vi "main_file.vi"() -> ()   [LabVIEW 2015]
uses:
  support VIs/User Event - Stop/User Event - Stop.lvlib
  support VIs/Message Queue/Message Queue.lvlib
  support VIs/Message Queue/Enqueue Message (Single).vi
  Type Definitions/DLTS_user_inputs.ctl
  Type Definitions/Tabs.ctl
  Type Definitions/Technique_selector.ctl
panel:
  out "Tabs 2":T1
  in  "Tabs":T1
  out "Cluster 2":T2
  in  "DLTS user inputs":T3 {"Delay time (ms)" format="%#_4p"; "# Windows" format="%#_4p"; "min window length (ms)" format="%#_4p"; "Pulse width (ms)" format="%#_4p"}
  in  "Error In":errorcluster
  in  "Preferences Button":bool
  in  "Settings Button":bool
  in  "Technique selector":T4
  in  "File Path Control":path
  in  "Play Button":bool
  in  "Record Button":bool
  in  "Process Stop Button":bool
  in  "Stop Button":bool
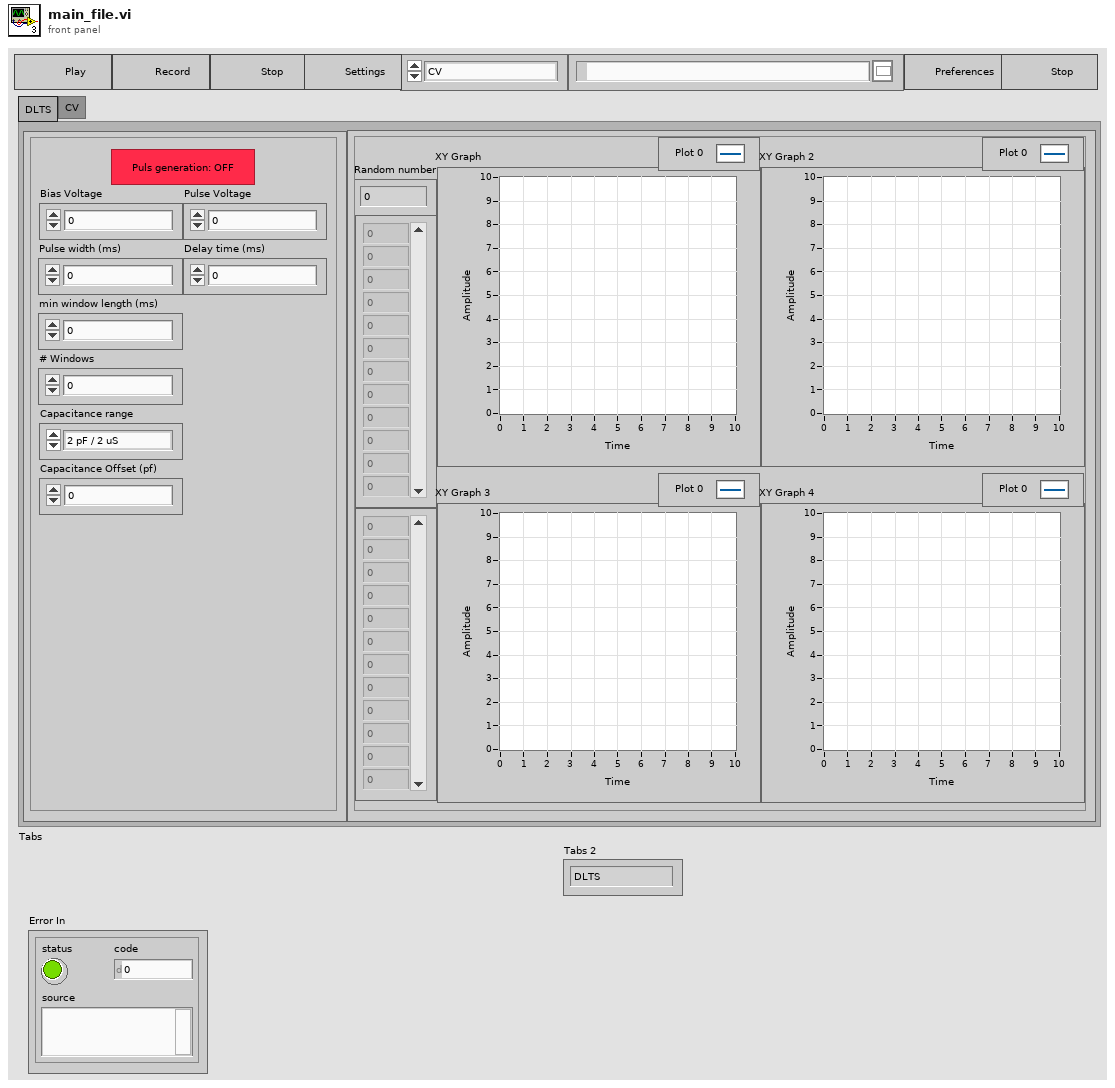
[diagram p1: front panel]
types:
  T1 = typedef "Tabs.ctl" = enum32{"DLTS", "CV"}
  T2 = cluster{"Array - Numeric 2":dbl[], "XY Graph":cluster{"X":dbl, "Y":dbl}[], "XY Graph 2":cluster{"X":dbl, "Y":dbl}[], "XY Graph 3":cluster{"X":dbl, "Y":dbl}[], "XY Graph 4":cluster{"X":dbl, "Y":dbl}[], "Array - Numeric":dbl[], "Random number":dbl}
  T3 = typedef "DLTS_user_inputs.ctl" = cluster{"Pulse Voltage":dbl, "Bias Voltage":dbl, "Pulse ON/OFF":bool, "Pulse width (ms)":dbl, "min window length (ms)":dbl, "# Windows":dbl, "Delay time (ms)":dbl, "Capacitance range":enum16{"2 pF / 2 uS", "20 pF / 20 uS", "200 pF / 200 uS", "2000 pF / 2000 uS"}, "Capacitance Offset (pf)":dbl}
  T4 = typedef "Technique_selector.ctl" = enum16{"CV", "IV", "DLTS"}
  T5 = typedef "Message Queue.lvlib/All Message Queues.ctl" = cluster{"UI":refnum<queue>, "CV Acquisition":refnum<queue>, "CV Logging":refnum<queue>, "IV Acquisition":refnum<queue>, "IV Logging":refnum<queue>, "DLTS Acquisiton":refnum<queue>, "DLTS Logging":refnum<queue>, "Acquisition":refnum<queue>, "Logging":refnum<queue>}
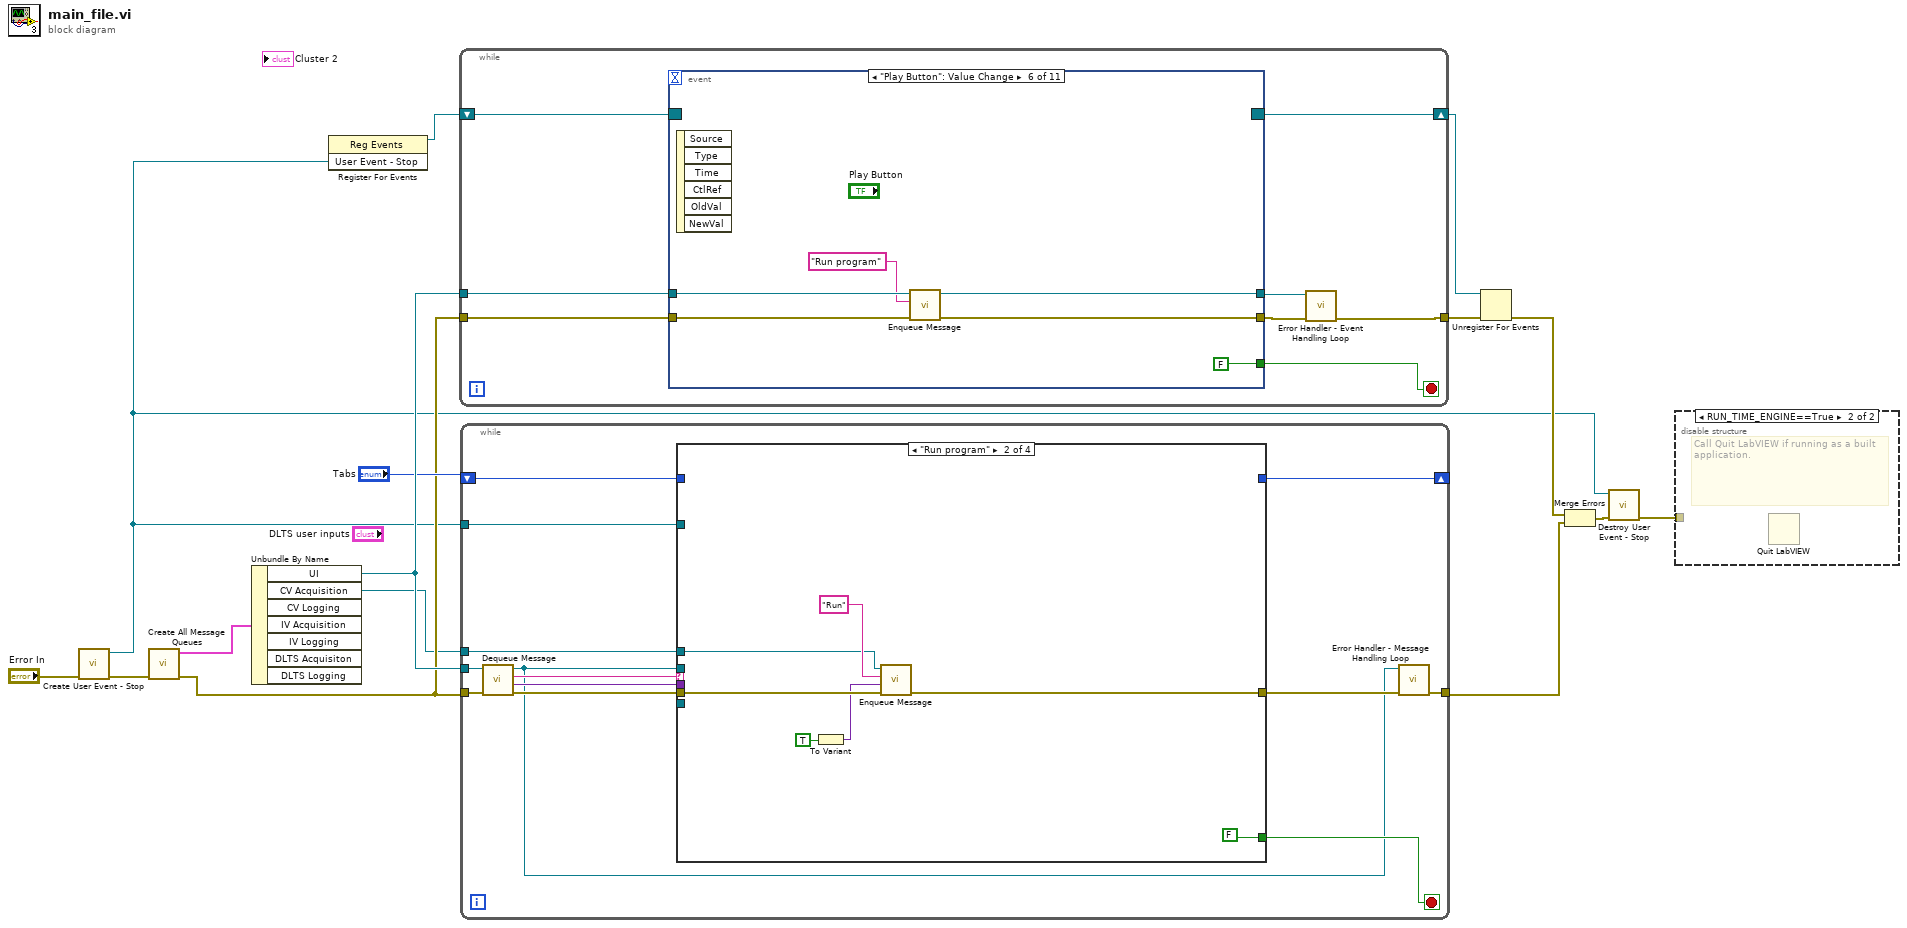
[diagram p0: block diagram]
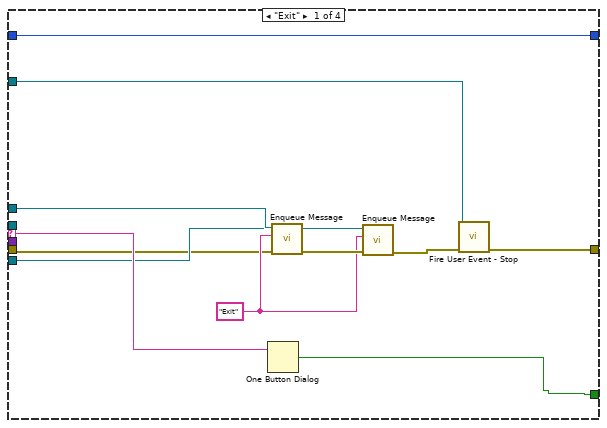
[diagram p3: hidden frame]
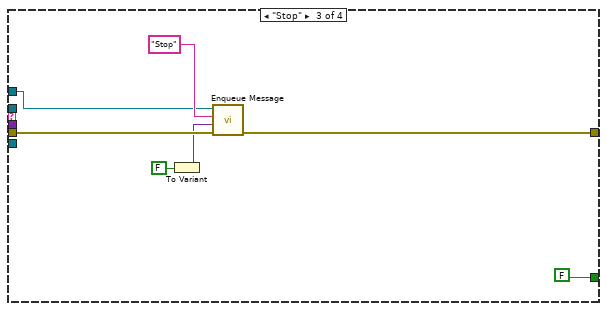
[diagram p4: hidden frame]
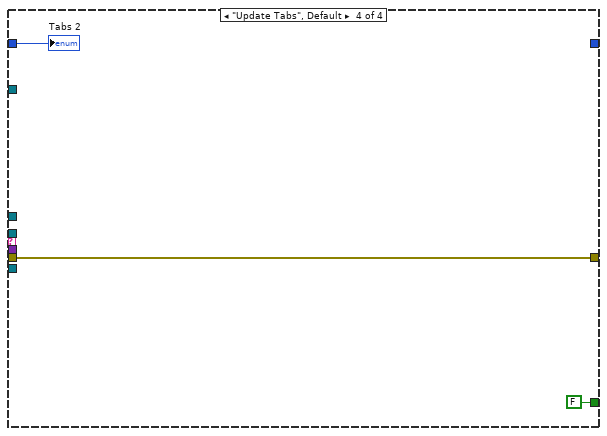
[diagram p5: hidden frame]
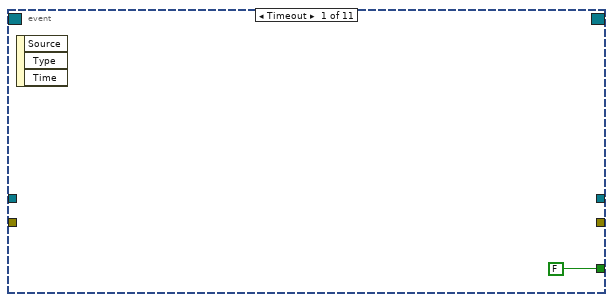
[diagram p6: hidden frame]
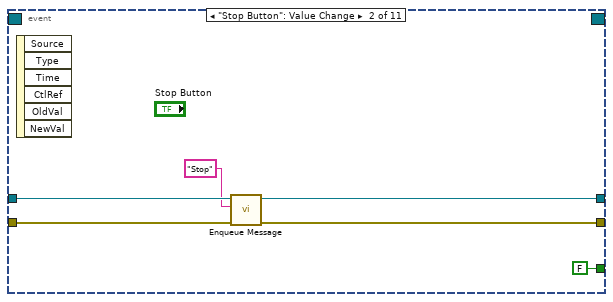
[diagram p7: hidden frame]
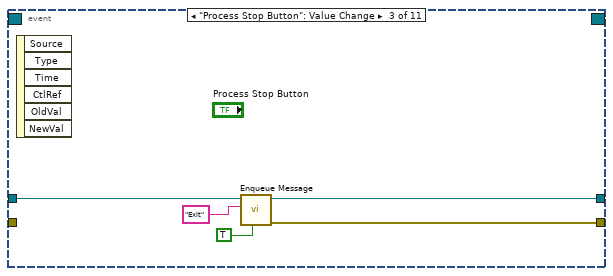
[diagram p8: hidden frame]
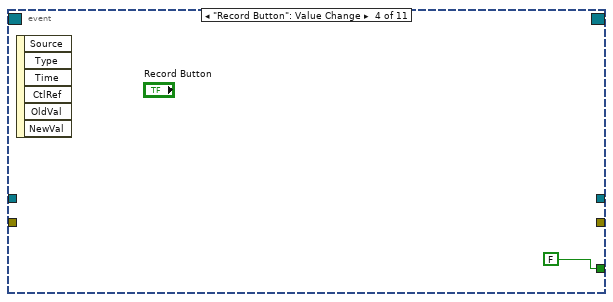
[diagram p9: hidden frame]
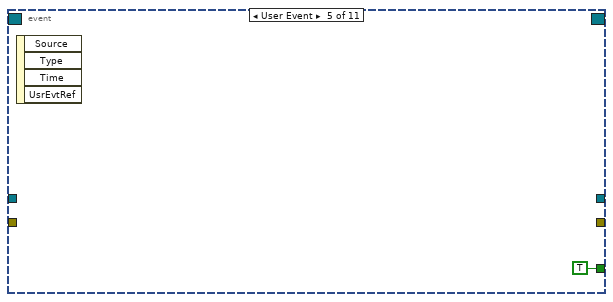
[diagram p10: hidden frame]
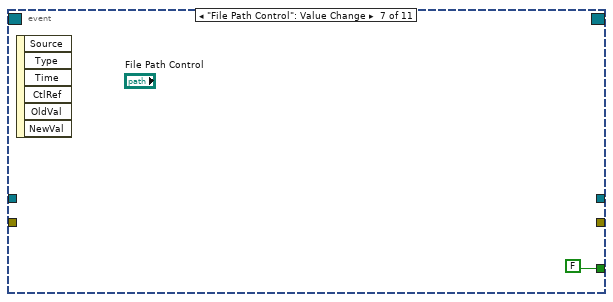
[diagram p11: hidden frame]
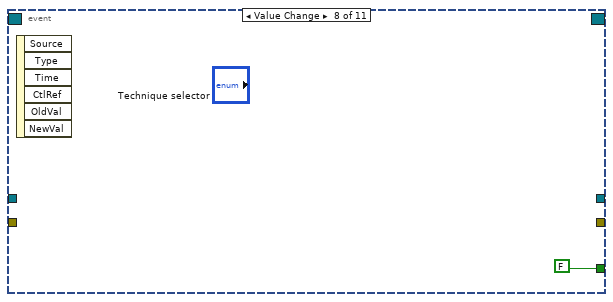
[diagram p12: hidden frame]
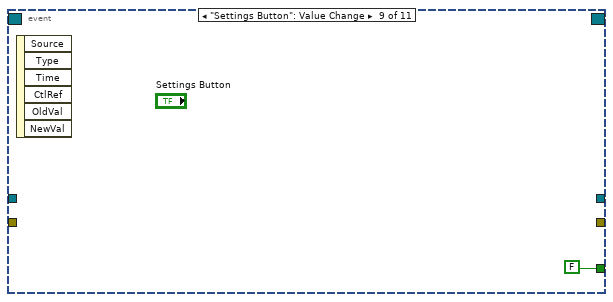
[diagram p13: hidden frame]
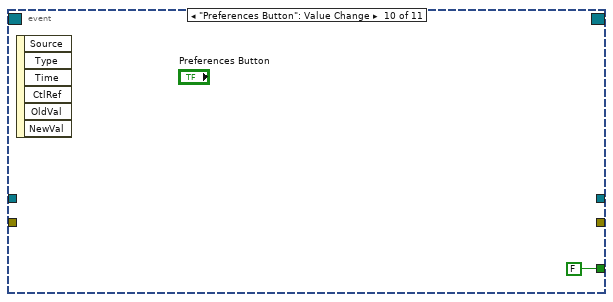
[diagram p14: hidden frame]
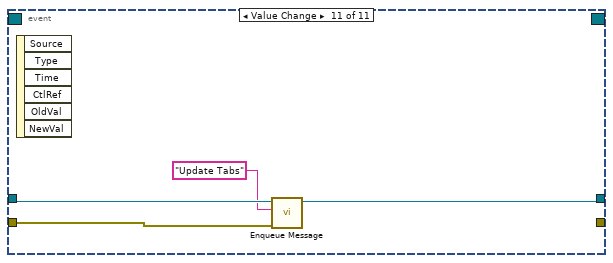
[diagram p15: hidden frame]
diagram:
  n1 = call "Create User Event - Stop.vi"("error in (no error)"="Error In") -> ("error out"=w13:errorcluster, "User Event - Stop"=w1:refnum<user-event>)  [unwired: 9 in]
  n2 = call "Create All Message Queues.vi"("error in (no error)"=w13) -> ("error out"=w4:errorcluster, "Message Queues out"=w3:T5)  [unwired: 9 in]
  n3 = Unbundle By Name(w3) -> ("UI"=w9:refnum<queue>, "CV Acquisition"=w2:refnum<queue>)  [unwired: 5 out]
  n4 = register-events(w1) -> (reference out=w12:refnum<event-registration>)  [unwired: 2 in, 1 out]
  n5 = while {
    shift-right: [w21] -> w10
    shift-left: w12 -> [w22]
    tunnel: w9 -> [w20]
    tunnel: [w17] -> w11
    tunnel: w4 -> [w19]
    stop <- w23 stop-if-true
    n6 = event shown="[5] \"Play Button\": Value Change" {
      selector: w22 -> [_ _ _ _ _ _ _ _ _ _ _]
      dyn-events: [_ _ _ _ _ _ _ _ _ _ _] -> w21
      timeout: _ -> [_ _ _ _ _ _ _ _ _ _ _]
      tunnel: [FALSE ("Process Stop Button") FALSE ("Process Stop Button") _ FALSE ("Process Stop Button") TRUE ("Process Stop Button") FALSE ("Process Stop Button") FALSE ("Process Stop Button") FALSE ("Process Stop Button") FALSE ("Process Stop Button") FALSE ("Process Stop Button") _] -> w23
      tunnel: w20 -> [_ w28 w35 _ _ w42 _ _ _ _ w50]
      tunnel: [_ w25 w34 _ _ w39 _ _ _ _ w51] -> w16
      tunnel: [_ w26 w33 _ _ w40 _ _ _ _ _] -> w18
      tunnel: w19 -> [_ w29 _ _ _ w41 _ _ _ _ w49]
      event Timeout {
        n7 = event-data() -> ()  [unwired: 1 in, 3 out]
      }
      event "Stop Button": Value Change {
        n8 = event-data() -> ()  [unwired: 1 in, 6 out]
        n9 = call-poly "Enqueue Message.vi"("error in (no error)"=w29, "Message"="Stop", "Message Queue"=w28) -> ("error out"=w26:errorcluster, "dup Message Queue"=w25:refnum<queue>)  [unwired: 7 in]
      }
      event "Process Stop Button": Value Change {
        n10 = event-data() -> ()  [unwired: 1 in, 6 out]
        n11 = call-poly "Enqueue Message.vi"("Priority Message? (F)"=TRUE, "Message"="Exit", "Message Queue"=w35) -> ("error out"=w33:errorcluster, "dup Message Queue"=w34:refnum<queue>)  [unwired: 7 in]
      }
      event "Record Button": Value Change {
        n12 = event-data() -> ()  [unwired: 1 in, 6 out]
      }
      event User Event {
        n13 = event-data() -> ()  [unwired: 1 in, 4 out]
      }
      event "Play Button": Value Change {
        n14 = event-data() -> ()  [unwired: 1 in, 6 out]
        n15 = call-poly "Enqueue Message.vi"("error in (no error)"=w41, "Message"="Run program", "Message Queue"=w42) -> ("error out"=w40:errorcluster, "dup Message Queue"=w39:refnum<queue>)  [unwired: 7 in]
      }
      event "File Path Control": Value Change {
        n16 = event-data() -> ()  [unwired: 1 in, 6 out]
      }
      event Value Change {
        n17 = event-data() -> ()  [unwired: 1 in, 6 out]
      }
      event "Settings Button": Value Change {
        n18 = event-data() -> ()  [unwired: 1 in, 6 out]
      }
      event "Preferences Button": Value Change {
        n19 = event-data() -> ()  [unwired: 1 in, 6 out]
      }
      event Value Change {
        n20 = event-data() -> ()  [unwired: 1 in, 6 out]
        n21 = call-poly "Enqueue Message.vi"("error in (no error)"=w49, "Message"="Update Tabs", "Message Queue"=w50) -> ("dup Message Queue"=w51:refnum<queue>)  [unwired: 7 in, 1 out]
      }
    }
    n22 = call "Error Handler - Event Handling Loop.vi"("error in (no error)"=w18, "Message Queue"=w16) -> ("dup error in"=w17:errorcluster)  [unwired: 8 in, 1 out]
  }
  n23 = while {
    tunnel: w9 -> [w64]
    tunnel: w4 -> [w60]
    shift-right: [w57] -> _
    shift-left: "Tabs" -> [w58]
    tunnel: w1 -> [w56]
    tunnel: [w54] -> w5
    tunnel: w2 -> [w55]
    stop <- w59 stop-if-true
    n24 = call "Dequeue Message.vi"("error in (no error)"=w60, "Message Queue"=w64) -> ("error out"=w61:errorcluster, "Message Data"=w62:variant, "Message"=w63:string, "dup Message Queue"=w52:refnum<queue>)  [unwired: 6 in]
    n25 = case shown="\"Run program\"" w63 {
      selector: w63 -> [w74 _ _ _]
      tunnel: w52 -> [_ _ _ _]
      tunnel: w62 -> [_ _ _ _]
      tunnel: w61 -> [w65 w82 w89 w90]
      tunnel: [w73 FALSE ("true") FALSE ("true") FALSE] -> w59
      tunnel: w58 -> [w75 _ _ w92]
      tunnel: [w75 _ _ _] -> w57
      tunnel: w56 -> [w72 _ _ _]
      tunnel: [w71 w80 w87 w90] -> w53
      tunnel: w55 -> [w68 w78 w85 _]
      tunnel: _ -> [w67 _ _ _]
      frame "Exit" {
        w66 = "Exit"
        n26 = One Button Dialog(message=w74) -> (true=w73:bool)  [unwired: 1 in]
        n27 = call-poly "Enqueue Message.vi"("error in (no error)"=w65, "Message"=w66, "Message Queue"=w68) -> ("error out"=w70:errorcluster)  [unwired: 7 in, 1 out]
        n28 = call-poly "Enqueue Message.vi"("error in (no error)"=w70, "Message"=w66, "Message Queue"=w67) -> ("error out"=w69:errorcluster)  [unwired: 7 in, 1 out]
        n29 = call "Fire User Event - Stop.vi"("error in (no error)"=w69, "User Event - Stop"=w72) -> ("error out"=w71:errorcluster)  [unwired: 9 in]
      }
      frame "Run program" {
        n30 = To Variant(anything=TRUE ("true")) -> (Variant=w76:variant)
        n31 = call-poly "Enqueue Message.vi"("error in (no error)"=w82, "Message Data"=w76, "Message"="Run", "Message Queue"=w78) -> ("error out"=w80:errorcluster)  [unwired: 6 in, 1 out]
      }
      frame "Stop" {
        n32 = To Variant(anything=FALSE ("true")) -> (Variant=w83:variant)
        n33 = call-poly "Enqueue Message.vi"("error in (no error)"=w89, "Message Data"=w83, "Message"="Stop", "Message Queue"=w85) -> ("error out"=w87:errorcluster)  [unwired: 6 in, 1 out]
      }
      frame "Update Tabs", Default {
        "Tabs 2" <- w92
      }
    }
    n34 = call "Error Handler - Message Handling Loop.vi"("error in (no error)"=w53, "Message Queue"=w52) -> ("dup error in"=w54:errorcluster)  [unwired: 8 in, 1 out]
  }
  n35 = Unregister For Events(event registration refnum=w10, error in=w11) -> (error out=w6:errorcluster)
  n36 = Merge Errors(w6, w5) -> (w7:errorcluster)
  n37 = call "Destroy User Event - Stop.vi"("error in (no error)"=w7, "User Event - Stop"=w1) -> ("error out"=w14:errorcluster)  [unwired: 9 in]
  n38 = disable-structure shown="RUN_TIME_ENGINE==True" {
    disable-tunnel: w14 -> [_ _]
    frame condition #0 (active) {
    }
    frame condition #1 {
      # "Call Quit LabVIEW if running as a built application."
      n39 = Quit LabVIEW() -> ()  [unwired: 1 in]
    }
  }
